vi "RT Host - calc distance travelled.vi"(8 "error in (no error)":errorcluster, 10 "Origin Global W/S Pos (mm)":dbl[](array[numeric])=[0.0, -90.0], 11 "From Global W/S Pos (mm)":dbl[](array[numeric])=[0.0, -90.0]) -> (0 "error out":errorcluster, 3 "Distance Travelled":dbl)   [LabVIEW 2017]
doc: "This subVI calculates the distance travelled from a given position."
panel:
  # "Inputs"
  # "Outputs"
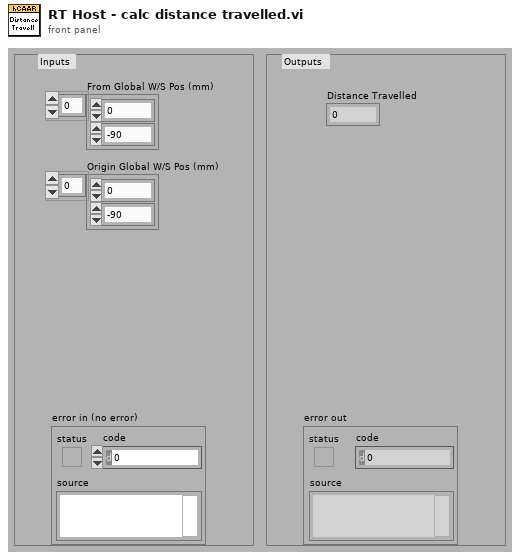
[diagram p1: front panel]
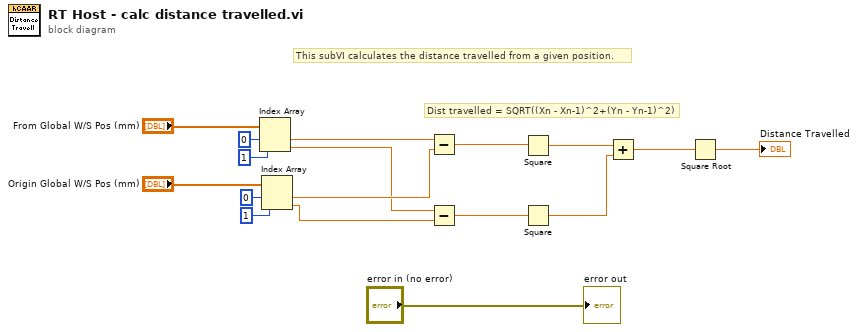
[diagram p0: block diagram]
diagram:
  # "This subVI calculates the distance travelled from a given position."
  # "Dist travelled = SQRT((Xn - Xn-1)^2+(Yn - Yn-1)^2)"
  n1 = Index Array(array="From Global W/S Pos (mm)", index #1=0 ("index"), index #2=1 ("index")) -> (element #1=w4:dbl, element #2=w3:dbl)
  n2 = Index Array(array="Origin Global W/S Pos (mm)", index #1=0 ("index"), index #2=1 ("index")) -> (element #1=w10:dbl, element #2=w11:dbl)
  n3 = Subtract(x=w4, y=w10) -> (x-y=w9:dbl)
  n4 = Subtract(x=w3, y=w11) -> (x-y=w8:dbl)
  n5 = Square(x=w9) -> (x^2=w12:dbl)
  n6 = Square(x=w8) -> (x^2=w13:dbl)
  n7 = Add(x=w12, y=w13) -> (x+y=w14:dbl)
  n8 = Square Root(x=w14) -> (sqrt(x)=→"Distance Travelled":dbl)
  "error out" <- "error in (no error)"
